vi "Remove State (from Connections).vi"(8 "error in (no error)":errorcluster, 10 "State":string, 11 "Channel Ref in":T1 format="%.0x") -> (0 "error out":errorcluster, 3 "Channel Ref out":T1=18446744073709551615 format="%.0x")   [LabVIEW 2017, in "Switch Scripting.lvlib"]
uses:
  Switch Scripting.lvlib
  <vilib>/NI Veristand/Custom Device API/Custom Device Item Ref.ctl
  NationalInstruments.VeriStand.SystemDefinitionAPI
  Shared/Constants.vi
  Shared/Switch Shared.lvlib
  <vilib>/NI VeriStand/Custom Device API/Custom Device API.lvlib
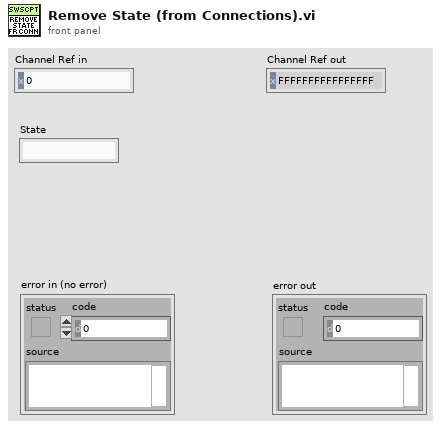
[diagram p1: front panel]
types:
  T1 = typedef "Custom Device API.lvlib/Custom Device Item Ref.ctl" = u64
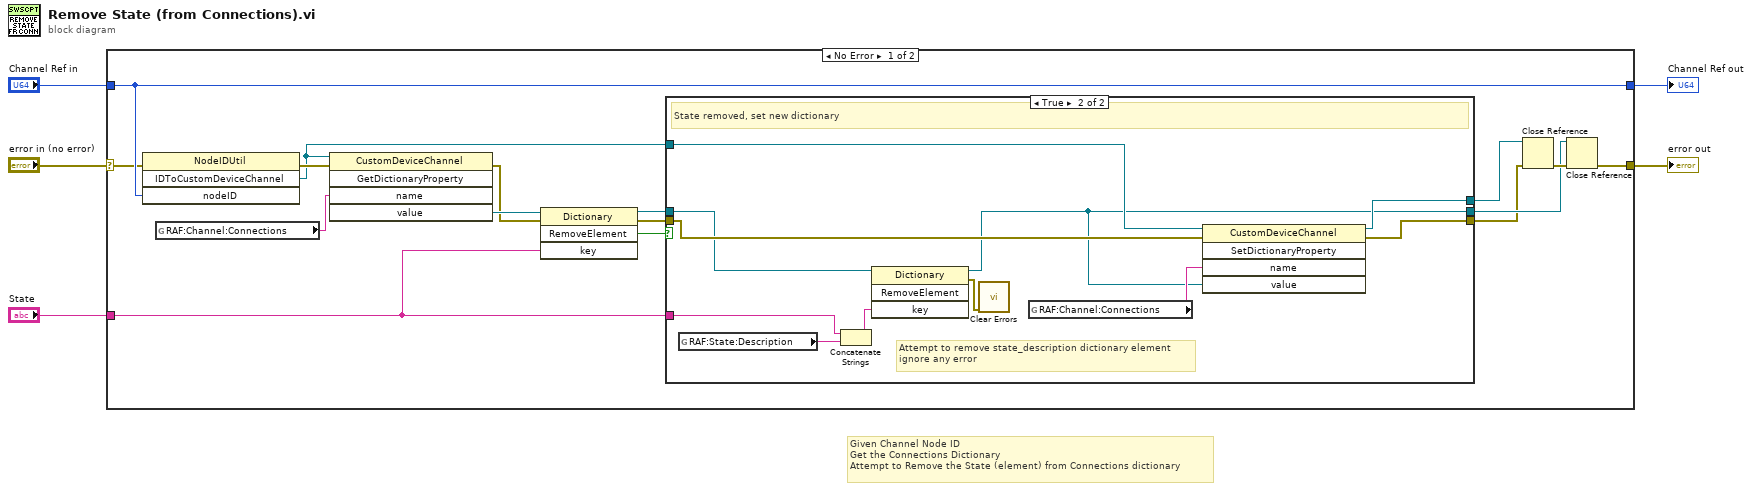
[diagram p0: block diagram]
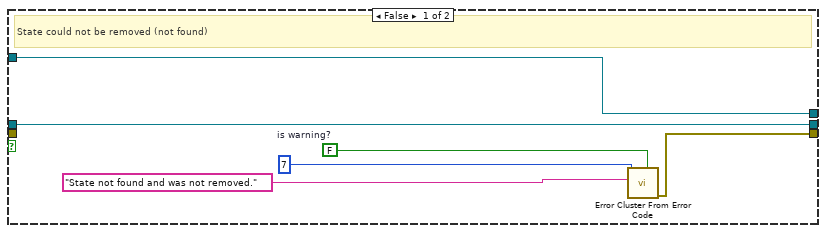
[diagram p2: hidden frame]
diagram:
  # "Given Channel Node ID\nGet the Connections Dictionary\nAttempt to Remove the State (element) from Connections dictionary"
  n1 = case shown="No Error" "error in (no error)" {
    selector: "error in (no error)" -> [w17 w40]
    tunnel: [w21 w40] -> w4
    tunnel: "Channel Ref in" -> [w18 w39]
    tunnel: [w18 w39] -> w2
    tunnel: "State" -> [w6 _]
    frame No Error {
      n2 = invoke class="NodeIDUtil" method="IDToCustomDeviceChannel"(error in=w17, "nodeID"=w18) -> (error out=w19:errorcluster, "IDToCustomDeviceChannel"=w9:refnum<k24>)  [unwired: 2 in, 2 out]
      n3 = global read "Constants.vi" "RAF:Channel:Connections"() -> (w7:string)
      n4 = invoke class="CustomDeviceChannel" method="GetDictionaryProperty"(reference=w9, error in=w19, "name"=w7) -> (error out=w15:errorcluster, "value"=w16:refnum<k24>)  [unwired: 2 in, 3 out]
      n5 = invoke class="Dictionary" method="RemoveElement"(reference=w16, error in=w15, "key"=w6) -> (reference out=w12:refnum<k24>, error out=w13:errorcluster, "RemoveElement"=w14:bool)  [unwired: 1 in, 1 out]
      n6 = case shown="True" w14 {
        tunnel: w13 -> [_ w38]
        tunnel: [w25 w37] -> w10
        tunnel: w12 -> [w24 w33]
        tunnel: [w24 w28] -> w11
        tunnel: w9 -> [w23 w36]
        tunnel: [w23 w35] -> w8
        tunnel: w6 -> [_ w31]
        frame False {
          w26 = FALSE  # is warning?
          # "State could not be removed (not found)"
          n7 = call <vilib>:"Error Cluster From Error Code.vi"("is warning? (False)"=w26, "error message (\"\")"="State not found and was not removed." ("error message (\"\")"), "error code (0)"=7) -> ("error out"=w25:errorcluster)  [unwired: 6 in]
        }
        frame True {
          # "Attempt to remove state_description dictionary element\nignore any error"
          # "State removed, set new dictionary"
          n8 = global read "Constants.vi" "RAF:State:Description"() -> (w32:string)
          n9 = Concatenate Strings(w31, w32) -> (w30:string)
          n10 = invoke class="Dictionary" method="RemoveElement"(reference=w33, "key"=w30) -> (reference out=w28:refnum<k24>, error out=w29:errorcluster)  [unwired: 2 in, 2 out]
          n11 = call <vilib>:"Clear Errors.vi"("error in (no error)"=w29) -> ()  [unwired: 5 in, 2 out]
          n12 = global read "Constants.vi" "RAF:Channel:Connections"() -> (w34:string)
          n13 = invoke class="CustomDeviceChannel" method="SetDictionaryProperty"(reference=w36, error in=w38, "name"=w34, "value"=w28) -> (reference out=w35:refnum<k24>, error out=w37:errorcluster)  [unwired: 1 in, 3 out]
        }
      }
      n14 = Close Reference(reference=w8, error in (no error)=w10) -> (error out=w20:errorcluster)
      n15 = Close Reference(reference=w11, error in (no error)=w20) -> (error out=w21:errorcluster)
    }
    frame Error {
    }
  }
  "Channel Ref out" <- w2
  "error out" <- w4
